vi "Get VI Images.vi"(8 "Error In":errorcluster, 10 "VI Path":path, 11 "Doc Config":T1) -> (0 "Error Out":errorcluster, 1 "BD_Img_Path":string, 2 "Con_Img_Path":string, 3 "Doc Config":T1)   [LabVIEW 2020, in "LMH-Toolbox.lvlib" / "LMH-Documentation.lvlib"]
uses:
  LMH-Documentation.lvlib
  Type Defs/Doc Config.ctl
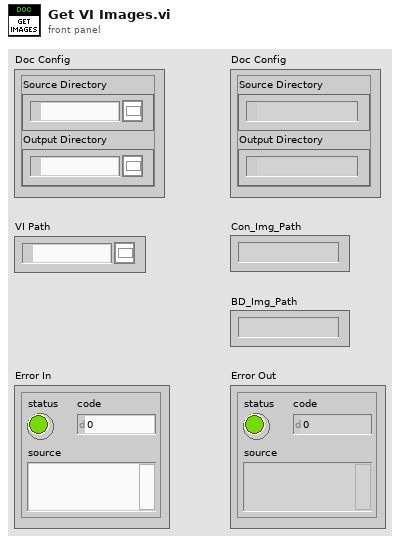
[diagram p1: front panel]
types:
  T1 = typedef "LMH-Toolbox.lvlib/LMH-Documentation.lvlib/Doc Config.ctl" = cluster{"Source Directory":path, "Output Directory":path}
  T2 = enum32{"Custom", "Standard", "Using Panel", "Using SubVI", "Complete"}
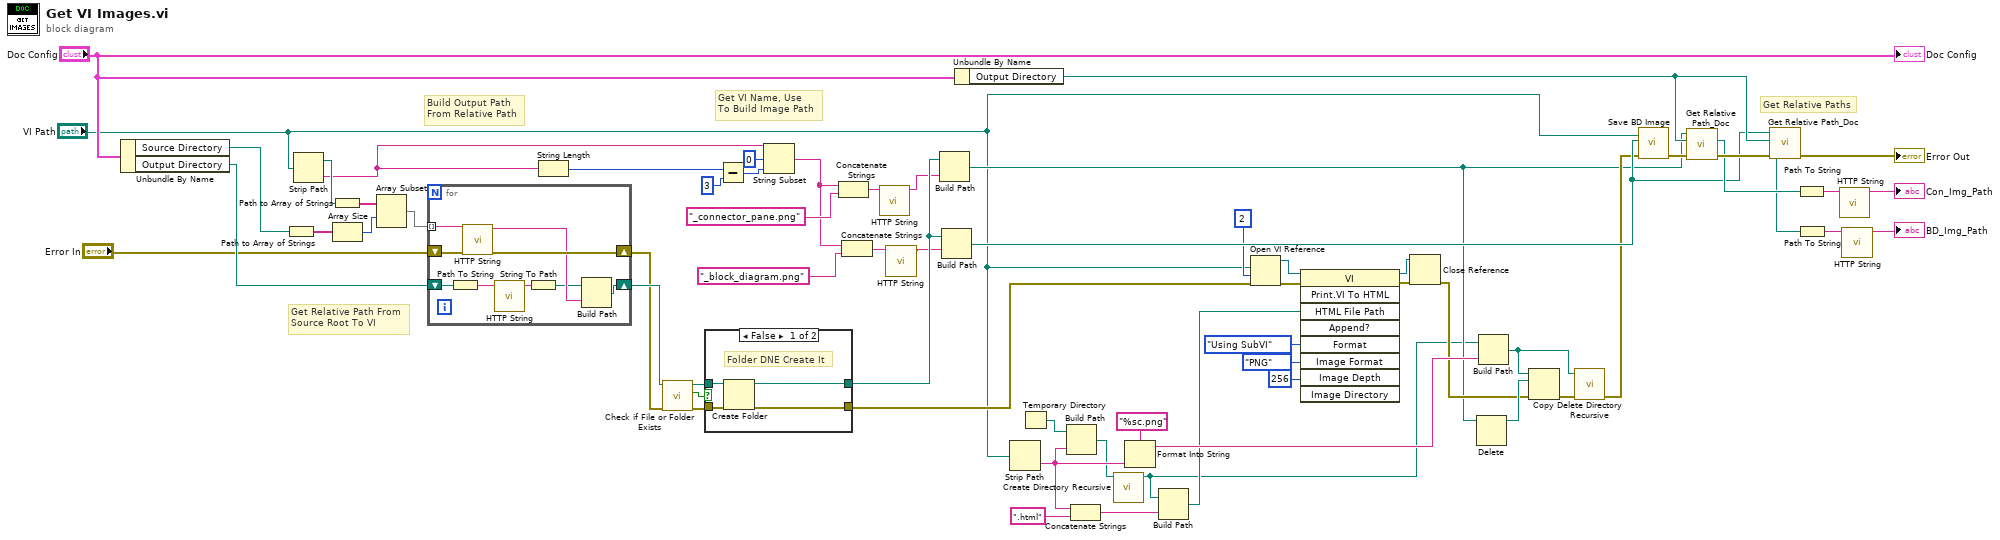
[diagram p0: block diagram]
diagram:
  # "Get Relative Paths"
  # "Get VI Name, Use \nTo Build Image Path"
  # "Build Output Path\nFrom Relative Path"
  # "Get Relative Path From\nSource Root To VI"
  n1 = Unbundle By Name("Doc Config") -> ("Source Directory"=w63:path, "Output Directory"=w62:path)
  n2 = Path to Array of Strings(0:w63) -> (2:w59:string[])  [unwired: 1 out]
  n3 = Strip Path(path="VI Path") -> (stripped path=w57:path, name=w56:string)
  n4 = Path to Array of Strings(0:w57) -> (2:w60:string[])  [unwired: 1 out]
  n5 = Array Size(array=w59) -> (size(s)=w61:i32)
  n6 = Array Subset(array=w60, index=w61) -> (w58:string[])  [unwired: 1 in]
  n7 = for {
    tunnel: w58 -> [w69] mode=indexing
    shift-right: [w72] -> w48
    shift-left: w62 -> [w66]
    shift-right: [w70] -> w31
    shift-left: "Error In" -> [w71]
    n8 = Path To String(path=w66) -> (string=w67:string)
    n9 = call "HTTP String.vi"("Error In"=w71, "String in"=w69) -> ("Error Out"=w70:errorcluster, "String out"=w68:string)  [unwired: 8 in]
    n10 = call "HTTP String.vi"("String in"=w67) -> ("String out"=w65:string)  [unwired: 9 in, 1 out]
    n11 = String To Path(string=w65) -> (path=w64:path)
    n12 = Build Path(base path=w64, name or relative path=w68) -> (appended path=w72:path)
  }
  n13 = String Length(string=w56) -> (length=w55:i32)
  n14 = call <vilib>:"Check if File or Folder Exists.vi"("error in (no error)"=w31, "path"=w48) -> ("error out"=w49:errorcluster, "file or folder exists?"=w50:bool, "dup path"=w51:path)  [unwired: 7 in]
  n15 = case shown="False" w50 {
    tunnel: [w74 w78] -> w20
    tunnel: w49 -> [w76 w78]
    tunnel: w51 -> [w75 w77]
    tunnel: [w73 w77] -> w43
    frame False {
      # "Folder DNE Create It"
      n16 = Create Folder(path (use dialog)=w75, error in=w76) -> (created path=w73:path, error out=w74:errorcluster)  [unwired: 1 in, 1 out]
    }
    frame True {
    }
  }
  n17 = Subtract(x=w55, y=3) -> (x-y=w53:i32)
  n18 = String Subset(string=w56, offset (0)=0, length (rest)=w53) -> (substring=w44:string)
  n19 = Concatenate Strings(w44, "_connector_pane.png" ("string")) -> (w29:string)
  n20 = Concatenate Strings(w44, "_block_diagram.png" ("string")) -> (w27:string)
  n21 = call "HTTP String.vi"("String in"=w29) -> ("String out"=w28:string)  [unwired: 9 in, 1 out]
  n22 = call "HTTP String.vi"("String in"=w27) -> ("String out"=w26:string)  [unwired: 9 in, 1 out]
  n23 = Build Path(base path=w43, name or relative path=w28) -> (appended path=w9:path)
  n24 = Build Path(base path=w43, name or relative path=w26) -> (appended path=w37:path)
  n25 = Unbundle By Name("Doc Config") -> ("Output Directory"=w40:path)
  n26 = Strip Path(path="VI Path") -> (name=w5:string)  [unwired: 1 out]
  n27 = Temporary Directory() -> (w4:path)
  n28 = Build Path(base path=w4, name or relative path=w5) -> (appended path=w3:path)
  n29 = Concatenate Strings(w5, ".html" ("string")) -> (w6:string)
  n30 = call <vilib>:"Create Directory Recursive.vi"("directory"=w3) -> ("directory copy"=w1:path)  [unwired: 4 in, 2 out]
  n31 = Format Into String(format string="%sc.png", w5) -> (resulting string=w11:string)  [unwired: 2 in, 1 out]
  n32 = Build Path(base path=w1, name or relative path=w6) -> (appended path=w2:path)
  n33 = Open VI Reference(vi path="VI Path", options=2, error in (no error)=w20) -> (vi reference=w24:refnum<vi>, error out=w23:errorcluster)  [unwired: 3 in]
  n34 = invoke class="VI" method="Print.VI To HTML"(reference=w24, error in=w23, "HTML File Path"=w2, "Format"=T2."Using SubVI", "Image Format"=enum32{"PNG", "JPEG", "GIF"}."PNG", "Image Depth"=256) -> (reference out=w21:refnum<vi>, error out=w22:errorcluster)  [unwired: 3 in, 7 out]
  n35 = Close Reference(reference=w21, error in (no error)=w22) -> (error out=w10:errorcluster)
  n36 = Delete(path (use dialog)=w9) -> (deleted path=w16:path)  [unwired: 4 in, 2 out]
  n37 = Build Path(base path=w1, name or relative path=w11) -> (appended path=w13:path)
  n38 = Copy(8:w10, 10:w16, 11:w13) -> (0:w15:errorcluster)  [unwired: 2 in, 2 out]
  n39 = call <vilib>:"Delete Directory Recursive.vi"("error in (no error)"=w15, "Folder to Delete"=w13) -> ("error out"=w14:errorcluster)  [unwired: 8 in, 1 out]
  n40 = call "Save BD Image.vi"("Error In"=w14, "Target BD Image Path"=w37, "VI Path"="VI Path") -> ("Error Out"=w42:errorcluster)  [unwired: 8 in]
  n41 = call "Get Relative Path_Doc.vi"("Error In"=w42, "Relative Path Root"=w40, "File / Folder"=w9) -> ("Error Out"=w41:errorcluster, "Relative Path"=w39:path)  [unwired: 6 in, 1 out]
  n42 = call "Get Relative Path_Doc.vi"("Error In"=w41, "Relative Path Root"=w40, "File / Folder"=w37) -> ("Error Out"=→"Error Out":errorcluster, "Relative Path"=w38:path)  [unwired: 6 in, 1 out]
  n43 = Path To String(path=w39) -> (string=w35:string)
  n44 = Path To String(path=w38) -> (string=w33:string)
  n45 = call "HTTP String.vi"("String in"=w35) -> ("String out"=→"Con_Img_Path":string)  [unwired: 9 in, 1 out]
  n46 = call "HTTP String.vi"("String in"=w33) -> ("String out"=→"BD_Img_Path":string)  [unwired: 9 in, 1 out]
  "Doc Config" <- "Doc Config"
